vi "AM FGV Data per Step.vi"(7 "CMD":T1, 8 "error in (no error)":errorcluster, 11 "Step Data in":dbl[](array[numeric])) -> (0 "error out":errorcluster, 3 "All Data out":dbl[](array[numeric]))   [LabVIEW 2020, in "Test Driver.lvlib"]
uses:
  Test Driver.lvlib
  support/PCT FGV CMD.ctl
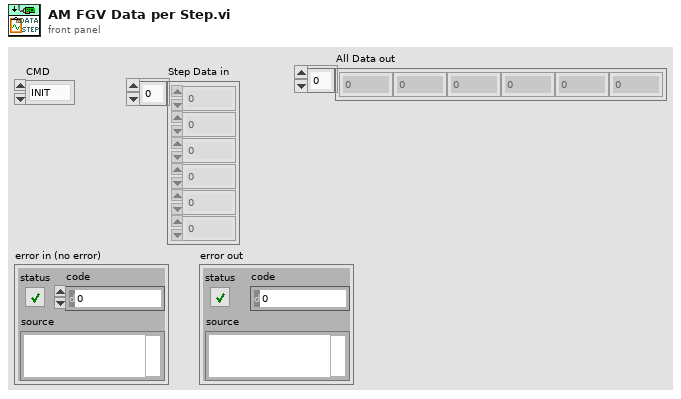
[diagram p1: front panel]
types:
  T1 = typedef "PCT FGV CMD.ctl" = enum16{"INIT", "GET", "SET"}
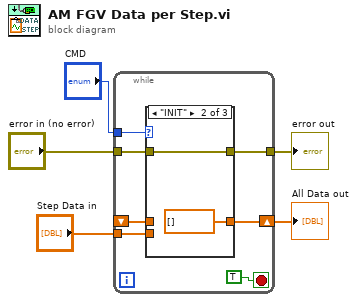
[diagram p0: block diagram]
diagram:
  n1 = while {
    tunnel: "CMD" -> [w10]
    shift-right: [w9] -> w5
    shift-left: _ -> [w8]
    tunnel: "error in (no error)" -> [w11]
    tunnel: [w12] -> w1
    tunnel: "Step Data in" -> [w6]
    stop <- TRUE stop-if-true
    n2 = case shown="\"INIT\"" w10 {
      tunnel: [w13 w16 w18] -> w12
      tunnel: [w14 dbl[] [] ("initialized array") w17] -> w9
      tunnel: w11 -> [w13 w16 w18]
      tunnel: w8 -> [w14 _ _]
      tunnel: w6 -> [_ _ w17]
      frame "GET", Default {
      }
      frame "INIT" {
      }
      frame "SET" {
      }
    }
  }
  "All Data out" <- w5
  "error out" <- w1
